vi "Generate Unhandled Step Error.vi"(8 "error in (no error)":errorcluster, 11 "Actor in":refnum<class "Actor.lvclass">) -> (0 "error out":errorcluster, 3 "Actor out":refnum<class "Actor.lvclass">)   [LabVIEW 2015, in "Actor.lvclass"]
uses:
  Actor.lvclass
  Actor.lvclass/Actor.ctl
  Sequencer/Sequencer.lvclass/Sequencer.ctl
  Sequencer/Sequencer.lvclass
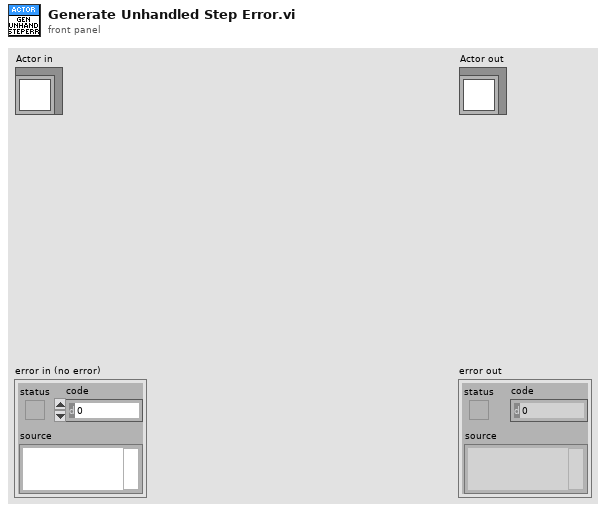
[diagram p1: front panel]
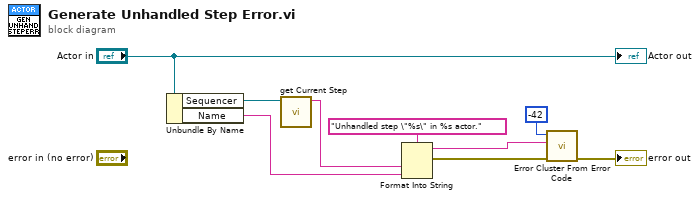
[diagram p0: block diagram]
diagram:
  n1 = Unbundle By Name("Actor in") -> ("Sequencer"=w4:refnum<class "Sequencer.lvclass">, "Name"=w5:string)
  n2 = call "get Current Step.vi"("Sequencer in"=w4) -> ("Current Step"=w1:string)  [unwired: 10 in]
  n3 = Format Into String(format string="Unhandled step \"%s\" in %s actor.", w1, w5) -> (resulting string=w2:string, error out=w7:errorcluster)  [unwired: 2 in]
  n4 = call <vilib>:"Error Cluster From Error Code.vi"("error in (no error)"=w7, "error message (\"\")"=w2, "error code (0)"=-42) -> ("error out"=→"error out":errorcluster)  [unwired: 6 in]
  "Actor out" <- "Actor in"
